vi "Set Lockout.vi"(0 "VISA resource name":refnum<visa-resource-name>, 1 "Unit Address (1)":i16=1, 5 "Action (0: Set Locks)":u16(ring) items=["Set Locks", "Clear Locks"], 7 "Access Levels (0; 0; 0; 0; 0; 0; 0)":u16[](array[ring])=[0, 0, 0, 0, 0, 0, 0] items=["Full Access", "Read Only", "Password", "Hidden"], 9 "Password (no text)":string, 11 "error in (no error)":errorcluster {"code" format="%.0x"}) -> (4 "VISA resource name out":refnum<visa-resource-name>, 15 "error out":errorcluster {"code" format="%.0x"})   [LabVIEW 2010]
doc: "This VI sets lockout and password."
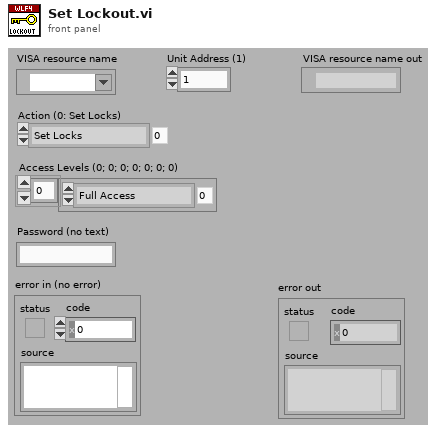
[diagram p1: front panel]
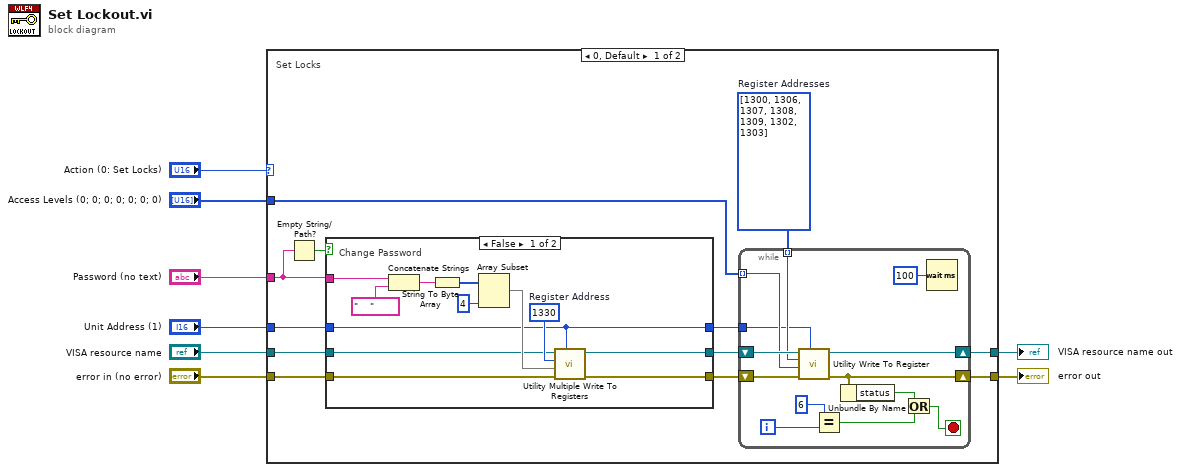
[diagram p0: block diagram]
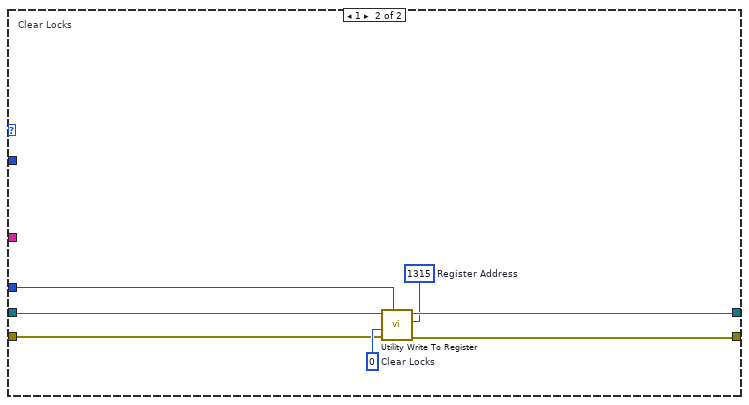
[diagram p3: hidden frame]
diagram:
  n1 = case shown="0, Default" "Action (0: Set Locks)" {
    tunnel: [w20 w55] -> w8
    tunnel: [w19 w54] -> w7
    tunnel: "Access Levels (0; 0; 0; 0; 0; 0; 0)" -> [w17 _]
    tunnel: "Password (no text)" -> [w10 _]
    tunnel: "Unit Address (1)" -> [w14 w49]
    tunnel: "VISA resource name" -> [w12 w50]
    tunnel: "error in (no error)" -> [w11 w51]
    frame 0, Default {
      w18 = i32[] [1300, 1306, 1307, 1308, 1309, 1302, 1303]  # Register Addresses
      # "Set Locks"
      n2 = Empty String/Path?(string/path=w10) -> (empty?=w9:bool)
      n3 = case shown="False" w9 {
        tunnel: w10 -> [w26 _]
        tunnel: [w22 w34] -> w16
        tunnel: [w23 w35] -> w15
        tunnel: w14 -> [w21 w33]
        tunnel: [w21 w33] -> w13
        tunnel: w12 -> [w25 w35]
        tunnel: w11 -> [w24 w34]
        frame False {
          w27 = u16 1330  # Register Address
          # "Change Password"
          n4 = Concatenate Strings(w26, "    " ("string")) -> (w30:string)
          n5 = String To Byte Array(string=w30) -> (unsigned byte array=w31:u8[])
          n6 = Array Subset(array=w31, length=4) -> (w29:u8[])  [unwired: 1 in]
          n7 = call "Utility Multiple Write To Registers.vi"("Unit Address (1)"=w21, "error in (no error)"=w24, "Array Of Data"=w29, "Register Address (0)"=w27, "VISA resource name"=w25) -> ("error out"=w22:errorcluster, "VISA resource name out"=w23:refnum<visa-resource-name>)  [unwired: 5 in]
        }
        frame True {
          # "No Change"
        }
      }
      n8 = while {
        shift-right: [w46] -> w19
        shift-left: w15 -> [w48]
        shift-right: [w44] -> w20
        shift-left: w16 -> [w47]
        tunnel: w17 -> [w43] mode=indexing
        tunnel: w18 -> [w38] mode=indexing
        tunnel: w13 -> [w36]
        i -> [w42]
        stop <- w41 stop-if-true
        n9 = call "Utility Write To Register.vi"("Unit Address (1)"=w36, "error in (no error)"=w47, "Data (0)"=w43, "Register Address (0)"=w38, "VISA resource name"=w48) -> ("error out"=w44:errorcluster, "VISA resource name out"=w46:refnum<visa-resource-name>)  [unwired: 5 in]
        n10 = Equal?(x=u32 6 ("milliseconds to wait"), y=w42) -> (x = y?=w40:bool)
        n11 = Unbundle By Name(w44) -> ("status"=w39:bool)
        n12 = Or(x=w39, y=w40) -> (x .or. y?=w41:bool)
        n13 = Wait (ms)(milliseconds to wait=u32 100) -> ()  [unwired: 1 out]
      }
    }
    frame 1 {
      w52 = i16 0  # Clear Locks
      w53 = u16 1315  # Register Address
      # "Clear Locks"
      n14 = call "Utility Write To Register.vi"("Unit Address (1)"=w49, "error in (no error)"=w51, "Data (0)"=w52, "Register Address (0)"=w53, "VISA resource name"=w50) -> ("error out"=w55:errorcluster, "VISA resource name out"=w54:refnum<visa-resource-name>)  [unwired: 5 in]
    }
  }
  "error out" <- w8
  "VISA resource name out" <- w7
